vi "Handle Last Ack Core.vi"(4 "error in (no error)":errorcluster, 6 "Last Ack":refnum<class "Last Ack.lvclass">, 7 "IModel in":refnum<class "IModel.lvclass">) -> (0 "error out":errorcluster, 3 "IModel out":refnum<class "IModel.lvclass">)   [LabVIEW 2020, in "MVA Framework.lvlib" / "IModel.lvlib" / "IModel.lvclass"]
doc: "(<B>Filename</B>: Actor Framework.lvlib:Actor.lvclass:Handle Last Ack Core.vi)\n\nDefines how the caller actor responds to the Last Ack message from a nested actor. The Last Ack message is the final message a nested actor sends to its caller before it shuts down. The message contains information about the final state of the nested actor.\n\nBy default, this method does nothing except return any error the nested actor sent. A descendant class may override this method to define behavior."
uses:
  IModel.lvclass
  <vilib>/ActorFramework/LastAck/Last Ack.lvclass
  C:/Program Files/National Instruments/LabVIEW 2020/vi.lib/ActorFramework/Actor/Actor.lvclass
  <vilib>/ActorFramework/LastAck/Last Ack.lvclass/Last Ack.ctl
  <vilib>/ActorFramework/Message/Message.lvclass
  IObserver/IObserver/IObserver.lvclass/IObserver.ctl
  composed-event-logger/Source/Composed Log/LoggerReference/LoggerReference.lvclass/LoggerReference.ctl
  IModel.lvclass/IModel.ctl
  <vilib>/ActorFramework/Actor/Actor.lvclass/Actor.ctl
  <vilib>/ActorFramework/Message Enqueuer/Message Enqueuer.lvclass/Message Enqueuer.ctl
  composed-event-logger/Source/Composed Log/LoggerReference/Log Event.vi
  <vilib>/ActorFramework/Actor/Read Self Enqueuer.vi
  <vilib>/ActorFramework/Message Enqueuer/Enqueue.vi
  composed-event-logger/Source/Composed Log/LoggerReference/Log.vi
  composed-event-logger/Source/Composed Log/LoggerReference/Get Valid Event Time.vi
  <vilib>/ActorFramework/Message Enqueuer/Init from Existing Queue.vi
  composed-event-logger/Source/Composed Log/LoggerReference/Remove Stale Logs.vi
  <vilib>/ActorFramework/Message Priority Queue/Priority Enqueue.vi
  <vilib>/ActorFramework/Message Enqueuer/Message Enqueuer.lvclass
  IObserver/IObserver/IObserver.lvclass
  <vilib>/ActorFramework/Actor/Actor.lvclass
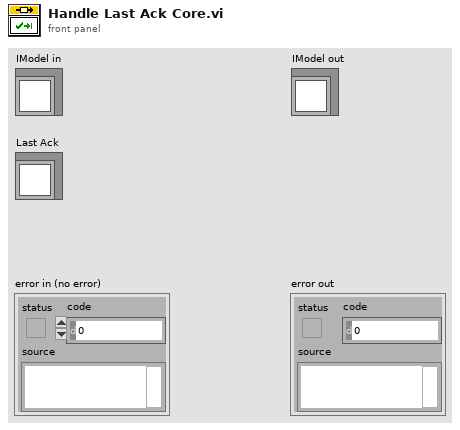
[diagram p1: front panel]
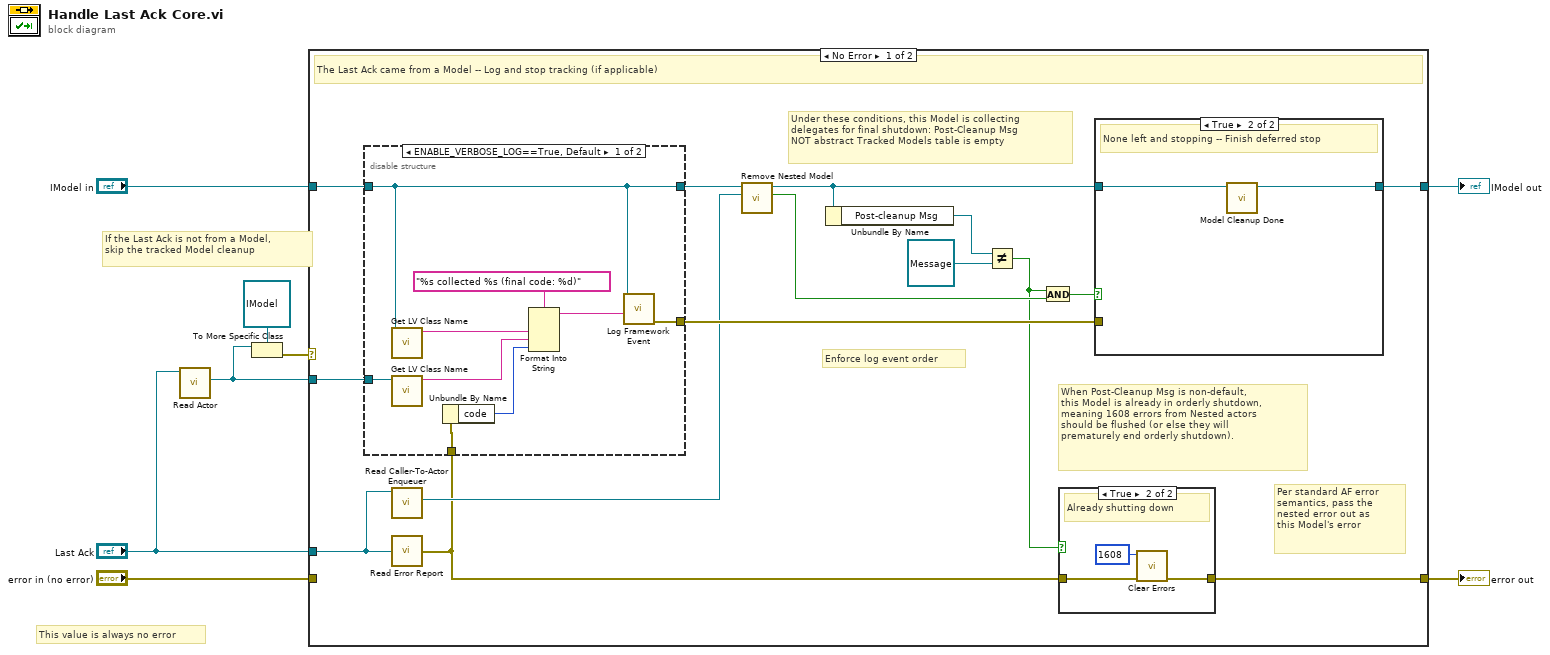
[diagram p0: block diagram]
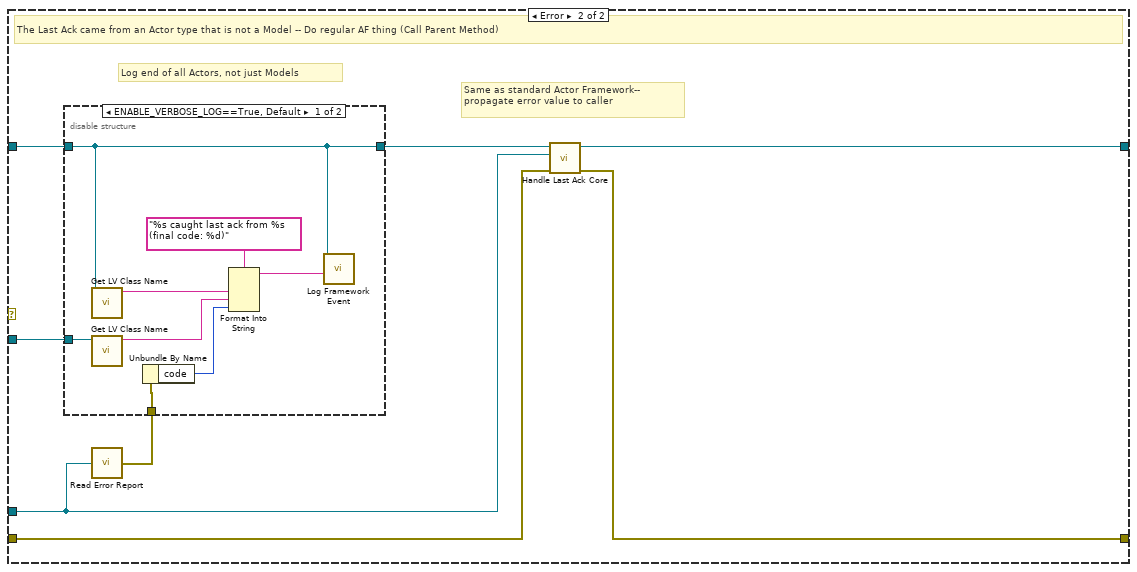
[diagram p5: hidden frame]
diagram:
  # "If the Last Ack is not from a Model,\nskip the tracked Model cleanup"
  # "This value is always no error"
  n1 = call <vilib>:"Read Actor.vi"("Last Ack"="Last Ack") -> ("Actor"=w1:refnum<class "Actor.lvclass">)  [unwired: 10 in]
  n2 = To More Specific Class(target class=refnum<class "IModel.lvclass"> refnum ("IModel.lvlib:IModel.lvclass"), reference=w1) -> (error out=w3:errorcluster)  [unwired: 1 in, 1 out]
  n3 = case shown="No Error" w3 {
    tunnel: "Last Ack" -> [w13 w43]
    tunnel: [w23 w48] -> w7
    tunnel: "IModel in" -> [w22 w45]
    tunnel: [w10 w46] -> w5
    tunnel: w1 -> [w20 w41]
    tunnel: "error in (no error)" -> [_ w47]
    frame No Error {
      # "Per standard AF error\nsemantics, pass the\nnested error out as\nthis Model's error"
      # "Enforce log event order"
      # "Under these conditions, this Model is collecting\ndelegates for final shutdown: Post-Cleanup Msg\nNOT abstract Tracked Models table is empty"
      # "The Last Ack came from a Model -- Log and stop tracking (if applicable)"
      # "When Post-Cleanup Msg is non-default,\nthis Model is already in orderly shutdown,\nmeaning 1608 errors from Nested actors\nshould be flushed (or else they will\nprematurely end orderly shutdown)."
      n4 = call <vilib>:"Read Caller-To-Actor Enqueuer.vi"("Last Ack"=w13) -> ("Caller-to-Actor Enqueuer"=w14:refnum<class "Message Enqueuer.lvclass">)  [unwired: 10 in]
      n5 = call <vilib>:"Read Error Report.vi"("Last Ack"=w13) -> ("error report"=w11:errorcluster)
      n6 = disable-structure shown="ENABLE_VERBOSE_LOG==True, Default" {
        disable-tunnel: [w34 _] -> w15
        disable-tunnel: w22 -> [w33 w37]
        disable-tunnel: [w33 w37] -> w21
        disable-tunnel: w20 -> [w30 _]
        disable-tunnel: w11 -> [w28 _]
        frame condition #0 (active) {
          # "Log Last Ack event"
          n7 = call <vilib>:"Get LV Class Name.vi"("object"=w33) -> ("class name"=w36:string)  [unwired: 9 in, 1 out]
          n8 = call <vilib>:"Get LV Class Name.vi"("object"=w30) -> ("class name"=w29:string)  [unwired: 9 in, 1 out]
          n9 = Unbundle By Name(w28) -> ("code"=w31:i32)
          n10 = Format Into String(format string="%s collected %s (final code: %d)", w36, w29, w31) -> (resulting string=w35:string)  [unwired: 2 in, 1 out]
          n11 = call "Log Framework Event.vi"("Data To Log"=w35, "IObserver in"=w33) -> ("error out"=w34:errorcluster)  [unwired: 9 in]
        }
        frame condition #1 {
          # "Remove all logging from this method at compile time"
        }
      }
      n12 = call "Remove Nested Model.vi"("Nested Model Enqueuer"=w14, "IModel in"=w21) -> ("None Remaining?"=w17:bool, "IModel out"=w12:refnum<class "IModel.lvclass">)  [unwired: 8 in]
      n13 = Unbundle By Name(w12) -> ("Post-cleanup Msg"=w18:refnum<class "Message.lvclass">)
      n14 = Not Equal?(x=w18, y=refnum<class "Message.lvclass"> refnum) -> (x != y?=w9:bool)
      n15 = And(x=w9, y=w17) -> (x .and. y?=w16:bool)
      n16 = case shown="True" w9 {
        tunnel: w11 -> [w24 w27]
        tunnel: [w24 w26] -> w10
        frame False {
          # "Not shutting down"
        }
        frame True {
          # "Already shutting down"
          n17 = call <vilib>:"Clear Errors.vi"("error in (no error)"=w27, "specific error code to clear (0: all)"=1608) -> ("error out"=w26:errorcluster)  [unwired: 4 in, 1 out]
        }
      }
      n18 = case shown="True" w16 {
        tunnel: w12 -> [w38 w39]
        tunnel: [w38 w40] -> w23
        tunnel: w15 -> [_ _]
        frame False {
          # "Keep waiting for last acks"
        }
        frame True {
          # "None left and stopping -- Finish deferred stop"
          n19 = call "Model Cleanup Done.vi"("IModel in"=w39) -> ("IModel out"=w40:refnum<class "IModel.lvclass">)  [unwired: 10 in]
        }
      }
    }
    frame Error {
      # "Log end of all Actors, not just Models"
      # "Same as standard Actor Framework--\npropagate error value to caller"
      # "The Last Ack came from an Actor type that is not a Model -- Do regular AF thing (Call Parent Method)"
      n20 = call <vilib>:"Read Error Report.vi"("Last Ack"=w43) -> ("error report"=w42:errorcluster)
      n21 = disable-structure shown="ENABLE_VERBOSE_LOG==True, Default" {
        disable-tunnel: w45 -> [w54 w57]
        disable-tunnel: [w54 w57] -> w44
        disable-tunnel: w41 -> [w51 _]
        disable-tunnel: w42 -> [w49 _]
        frame condition #0 (active) {
          # "Log Last Ack event"
          n22 = call <vilib>:"Get LV Class Name.vi"("object"=w54) -> ("class name"=w56:string)  [unwired: 9 in, 1 out]
          n23 = call <vilib>:"Get LV Class Name.vi"("object"=w51) -> ("class name"=w50:string)  [unwired: 9 in, 1 out]
          n24 = Unbundle By Name(w49) -> ("code"=w52:i32)
          n25 = Format Into String(format string="%s caught last ack from %s (final code: %d)", w56, w50, w52) -> (resulting string=w55:string)  [unwired: 2 in, 1 out]
          n26 = call "Log Framework Event.vi"("Data To Log"=w55, "IObserver in"=w54) -> ()  [unwired: 9 in, 1 out]
        }
        frame condition #1 {
          # "Remove all logging from this method at compile time"
        }
      }
      n27 = call-parent "Handle Last Ack Core.vi"("error in (no error)"=w47, "Last Ack"=w43, "Actor in"=w44) -> ("error out"=w46:errorcluster, "Actor out"=w48:refnum<class "IModel.lvclass">)  [unwired: 3 in]
    }
  }
  "IModel out" <- w7
  "error out" <- w5
